vi "Verify Voltage.vi"(8 "error in":errorcluster, 11 "6700 in":refnum<class "6700.lvclass">) -> (0 "error out":errorcluster, 3 "6700 out":refnum<class "6700.lvclass">)   [LabVIEW 2018, in "6700.lvlib" / "6700.lvclass"]
uses:
  6700.lvclass
  6700.lvclass/6700.ctl
  builds/Power_Supply.lvlibp/Power Supply.lvclass
  C:/Users/Ron.Dexter.LUMINARTECH/Desktop/builds/Power_Supply.lvlibp/Power Supply.lvclass
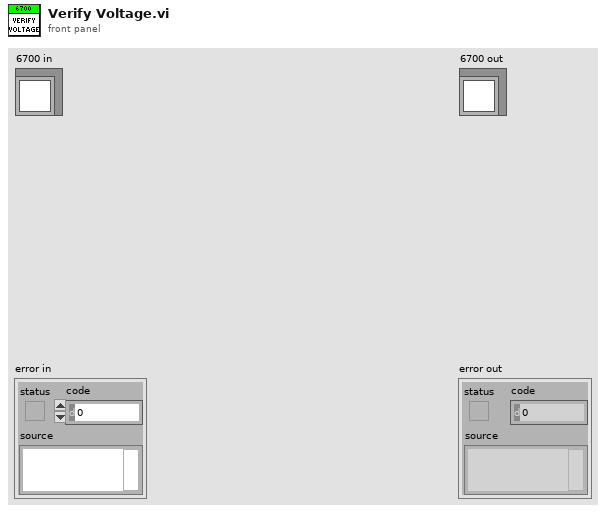
[diagram p1: front panel]
types:
  T1 = typedef "Power_Supply.lvlibp/Supply Settings.ctl" = cluster{"Voltage":dbl, "Current":dbl, "Output":bool}
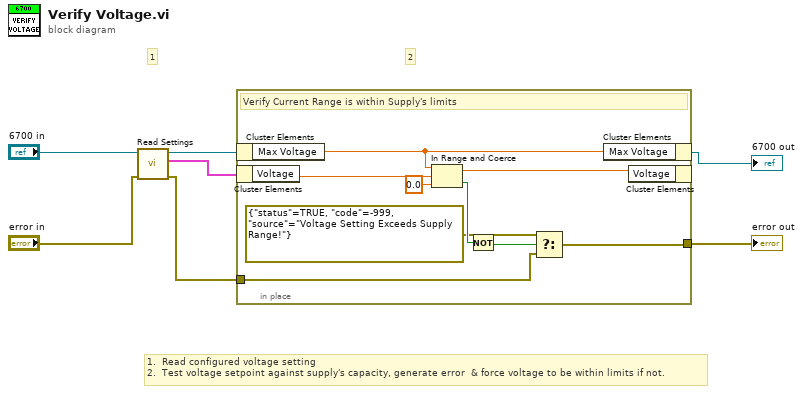
[diagram p0: block diagram]
diagram:
  # "1.  Read configured voltage setting\n2.  Test voltage setpoint against supply's capacity, generate error  & force voltage to be within limits if not."
  # "2"
  # "1"
  n1 = call "Read Settings.vi"("error in (no error)"="error in", "Power Supply in"="6700 in") -> ("error out"=w3:errorcluster, "Settings"=w4:T1, "Power Supply out"=w5:refnum<class "6700.lvclass">)  [unwired: 7 in]
  n2 = in-place {
    in-place-border: w3 -> [w11]
    in-place-border: [w10] -> w1
    # "Verify Current Range is within Supply's limits"
    n3 = in-place-cluster #1(w5) -> ("Max Voltage"=w16:dbl)
    n4 = in-place-cluster #2(w4) -> ("Voltage"=w15:dbl)
    n5 = In Range and Coerce(upper limit=w16, x=w15, lower limit=0.0) -> (coerced(x)=w14:dbl, In Range?=w13:bool)
    n6 = Not(x=w13) -> (.not. x?=w12:bool)
    n7 = Select(t=errorcluster {"status"=TRUE, "code"=-999, "source"="Voltage Setting Exceeds Supply Range!"} ("error out"), s=w12, f=w11) -> (s? t:f=w10:errorcluster)
    n8 = in-place-cluster #1("Max Voltage"=w16) -> (→"6700 out":refnum<class "6700.lvclass">)
    n9 = in-place-cluster #2("Voltage"=w14) -> ()  [unwired: 1 out]
  }
  "error out" <- w1
